vi "Write Table Predefined infos.vi"(0 "PDF Table Class.lvclass in":refnum<class "Pdfp Table Class.lvclass">, 5 "Predefined Borders":T19={"Borders"=0, "Header"={"Thickness"=1.0, "Line"=0, "Background "=16777226}, "Data"={"Thickness"=0.5, "Line"=0, "Background "=16777215}}, 7 "Borders IN":T21, 9 "Column Header format":T18, 11 "error in (no error)":errorcluster, 12 "Row Header format":T18, 13 "Datas format":T18) -> (4 "PDF Table Class.lvclass out":refnum<class "Pdfp Table Class.lvclass">, 8 "Row  [ ] OUT":T1, 15 "error out":errorcluster)   [LabVIEW 2019, in "Pdfp Table Class.lvclass"]
uses:
  <userlib>/Exaprom PDF/LV Class/Pdfp Table Class/Pdfp Table Class.lvclass
  <userlib>/Exaprom PDF/Controls/Table Controls/Simplified Table Row Borders [ ].ctl
  <userlib>/Exaprom PDF/Controls/Table Controls/Simplified Table Row Borders.ctl
  <userlib>/Exaprom PDF/Controls/Table Controls/Border and BG Color [ ].ctl
  <userlib>/Exaprom PDF/Controls/Table Controls/Border and BG Color.ctl
  <userlib>/Exaprom PDF/Controls/Table Controls/Cell Border 20 px.ctl
  <userlib>/Exaprom PDF/Controls/Table Controls/Row Predefined borders cluster.ctl
  <userlib>/Exaprom PDF/Controls/Table Controls/Row Predefined borders.ctl
  <userlib>/Exaprom PDF/Controls/Table Controls/Cell Font, type, Alignment and LS V2.ctl
  <userlib>/Exaprom PDF/Controls/Table Controls/Cell Type, Alignment and LS.ctl
  <userlib>/Exaprom PDF/Controls/Table Controls/Cell Alignment 20px.ctl
  <userlib>/Exaprom PDF/Controls/Table Controls/Text vertical arrangement.ctl
  <userlib>/Exaprom PDF/Controls/Text Controls/Line spacing.ctl
  <userlib>/Exaprom PDF/Controls/Font Controls/Font complete cluster.ctl
  <userlib>/Exaprom PDF/Controls/Font Controls/Font size.ctl
  <userlib>/Exaprom PDF/Controls/Font Controls/Font color.ctl
  <userlib>/Exaprom PDF/Controls/Font Controls/Type and encoding.ctl
  <userlib>/Exaprom PDF/Controls/Text Controls/Unicode/Type and run direction.ctl
  <userlib>/Exaprom PDF/Controls/Table Controls/Table Appearance and Font Row [ ].ctl
  <userlib>/Exaprom PDF/Controls/Table Controls/One Row Appearance.ctl
  <userlib>/Exaprom PDF/Controls/Table Controls/Row from to.ctl
  <userlib>/Exaprom PDF/Controls/Table Controls/Cell, Alignment, LS and Font - hide Vmerge.ctl
  <userlib>/Exaprom PDF/Controls/Table Controls/Cell Appearance.ctl
  <userlib>/Exaprom PDF/Controls/Table Controls/Merge Horizontal.ctl
  <userlib>/Exaprom PDF/Controls/Table Controls/Merge Vertical.ctl
  <userlib>/Exaprom PDF/LV Class/Pdfp Table Class/Pdfp Table Class.lvclass/Pdfp Table Class.ctl
  <userlib>/Exaprom PDF/Controls/Table Controls/Table Custom type Titles or Datas.ctl
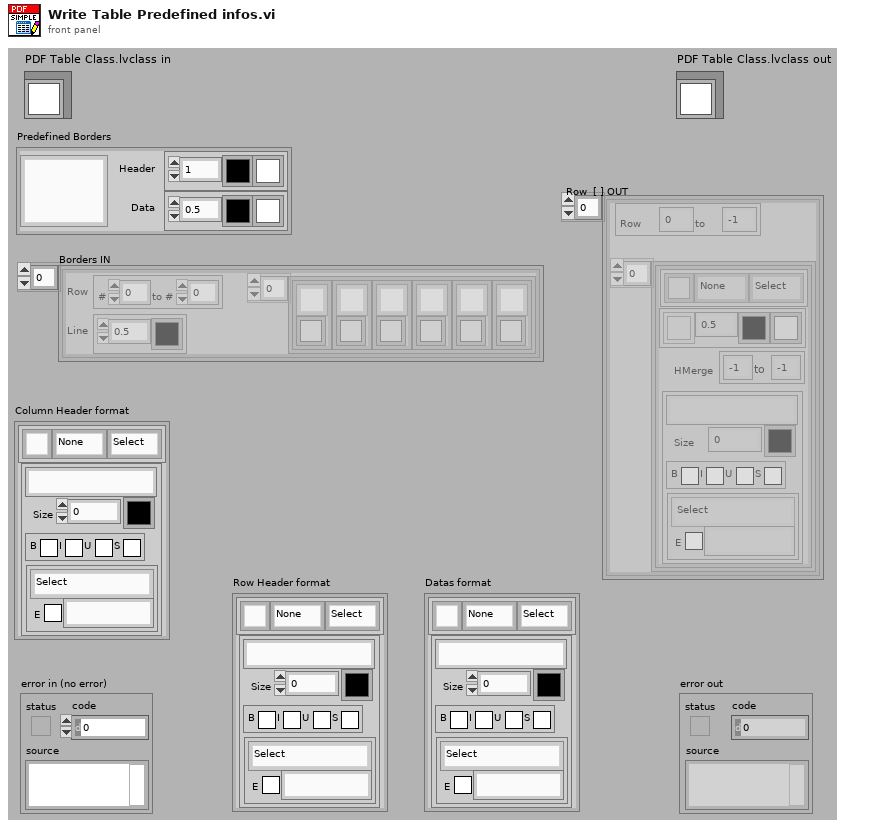
[diagram p1: front panel]
types:
  T1 = typedef "Table Appearance and Font Row [ ].ctl" = T2[]
  T2 = typedef "One Row Appearance.ctl" = cluster{"Row":T3, "Cell [ ]":T4[]}
  T3 = typedef "Row from to.ctl" = cluster{"From #":i16, "to #":i16}
  T4 = typedef "Cell, Alignment, LS and Font - hide Vmerge.ctl" = cluster{"Text":T5, "Cell Appearance":T9, "HMerge":T11, "VMerge":T12, "Font":T13}
  T5 = typedef "Cell Type, Alignment and LS.ctl" = cluster{"Cell Alignment":T6, "Text rotation":T7, "Line spacing":T8}
  T6 = typedef "Cell Alignment 20px.ctl" = u16
  T7 = typedef "Text vertical arrangement.ctl" = enum16{"None", "Clockwise", "Counterclockwise"}
  T8 = typedef "Line spacing.ctl" = enum16{"Select", "1.0", "1.5", "2.0"}
  T9 = typedef "Cell Appearance.ctl" = cluster{"Border":T10, "Thickness":sgl, "Color":u32, "BG":u32}
  T10 = typedef "Cell Border 20 px.ctl" = u16
  T11 = typedef "Merge Horizontal.ctl" = cluster{"From":i8, "to":i8}
  T12 = typedef "Merge Vertical.ctl" = cluster{"From":i8, "to":i8}
  T13 = typedef "Font complete cluster.ctl" = cluster{"Name":string, "Size":T14, "Color":T15, "Style":cluster{"Bold":bool, "Italic":bool, "Underline":bool, "Strikeout":bool}, "Type":T16}
  T14 = typedef "Font size.ctl" = sgl
  T15 = typedef "Font color.ctl" = u32
  T16 = typedef "Type and encoding.ctl" = cluster{"Type&direction":T17, "Embedded":bool, "Encoding":string}
  T17 = typedef "Type and run direction.ctl" = enum16{"Select", "ASCII", "UTF-16", "UTF-16 (default)", "UTF-16 (LTR)", "UTF-16 (RTL)"}
  T18 = typedef "Cell Font, type, Alignment and LS V2.ctl" = cluster{"Cell Type, Alignment and LS":T5, "Font":T13}
  T19 = typedef "Row Predefined borders cluster.ctl" = cluster{"Borders":T20, "Header":cluster{"Thickness":sgl, "Line":u32, "Background ":u32}, "Data":cluster{"Thickness":sgl, "Line":u32, "Background ":u32}}
  T20 = typedef "Row Predefined borders.ctl" = u16
  T21 = typedef "Simplified Table Row Borders [ ].ctl" = T22[]
  T22 = typedef "Simplified Table Row Borders.ctl" = cluster{"Row":cluster{"#":i16, "to #":i16}, "Line":cluster{"Thickness":sgl, "Color":u32}, "Column Borders [ ]":T23}
  T23 = typedef "Border and BG Color [ ].ctl" = T24[]
  T24 = typedef "Border and BG Color.ctl" = cluster{"Cell Border":T10, "BG":u32}
  T25 = typedef "Table Custom type Titles or Datas.ctl" = enum16{"Title", "Data"}
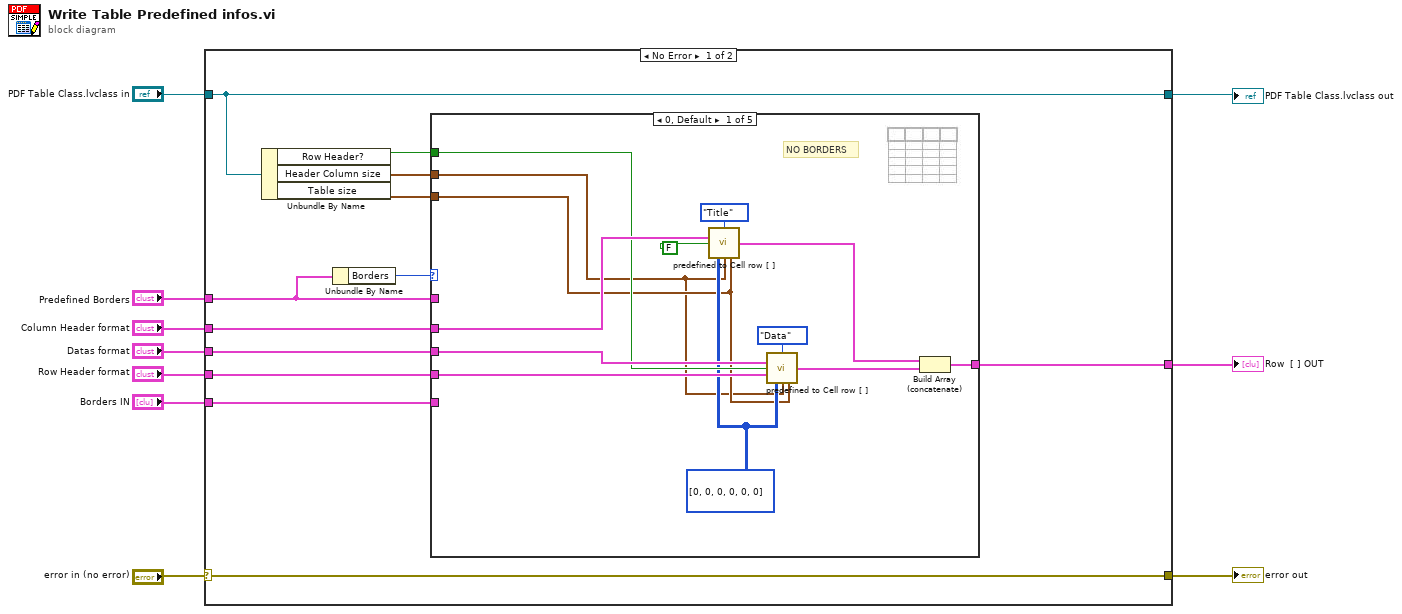
[diagram p0: block diagram]
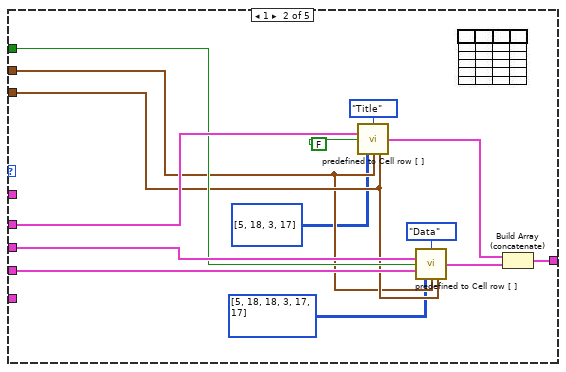
[diagram p2: hidden frame]
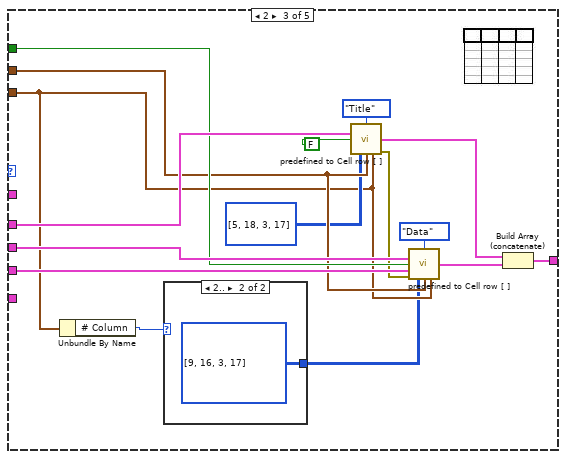
[diagram p3: hidden frame]
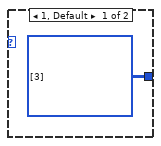
[diagram p4: hidden frame]
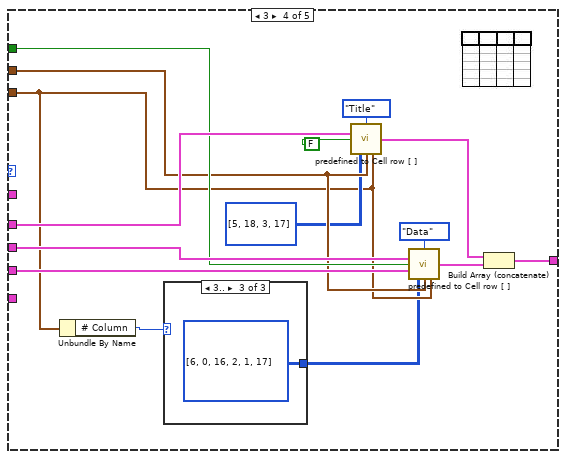
[diagram p5: hidden frame]
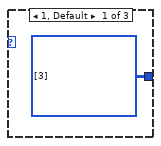
[diagram p6: hidden frame]
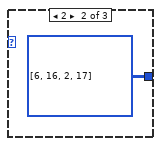
[diagram p7: hidden frame]
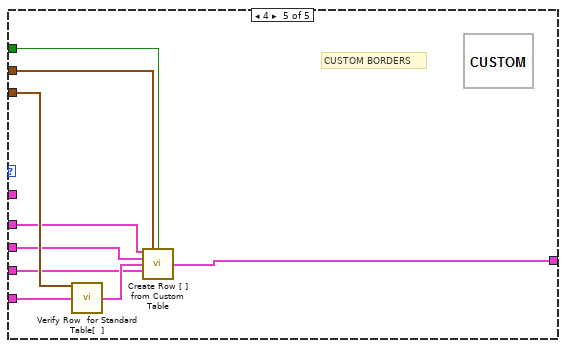
[diagram p8: hidden frame]
diagram:
  n1 = case shown="No Error" "error in (no error)" {
    selector: "error in (no error)" -> [w13 w96]
    tunnel: [w13 w96] -> w8
    tunnel: "Borders IN" -> [w22 _]
    tunnel: "Predefined Borders" -> [w21 _]
    tunnel: "PDF Table Class.lvclass in" -> [w12 w95]
    tunnel: [w12 w95] -> w5
    tunnel: "Column Header format" -> [w19 _]
    tunnel: "Row Header format" -> [w18 _]
    tunnel: "Datas format" -> [w17 _]
    tunnel: [w11 _] -> w1
    frame No Error {
      n2 = Unbundle By Name(w12) -> ("Row Header?"=w16:bool, "Header Column size"=w15:cluster{"# Column":u16, "# Row":u16}, "Table size"=w14:cluster{"# Column":u16, "# Row":u16})
      n3 = Unbundle By Name(w21) -> ("Borders"=w20:T20)
      n4 = case shown="0, Default" w20 {
        tunnel: w22 -> [_ _ _ _ w94]
        tunnel: w21 -> [_ _ _ _ _]
        tunnel: [w35 w49 w65 w82 w86] -> w11
        tunnel: w19 -> [w32 w46 w62 w79 w90]
        tunnel: w18 -> [w30 w44 w60 w77 w87]
        tunnel: w17 -> [w29 w43 w59 w76 w89]
        tunnel: w16 -> [w28 w42 w58 w75 w92]
        tunnel: w15 -> [w23 w38 w55 w72 w91]
        tunnel: w14 -> [w24 w39 w53 w70 w93]
        frame 0, Default {
          w27 = T10[][] [[0, 0, 0], [0, 0, 0]] ("Title tous 2")
          # "NO BORDERS"
          n5 = call <userlib>:"predefined to Cell row [ ].vi"("Titles or datas"=Table_Custom_type_Titles_or_Datas."Title", "Format Column Header or Data"=w32, "Row Header?"=FALSE, "Title tous"=w27, "Header Column size"=w23, "Table size"=w24) -> ("Row  [ ]"=w25:T1)  [unwired: 4 in, 5 out]
          n6 = call <userlib>:"predefined to Cell row [ ].vi"("Titles or datas"=Table_Custom_type_Titles_or_Datas."Data", "Format Column Header or Data"=w29, "Row Header?"=w28, "Format Row Header"=w30, "Title tous"=w27, "Header Column size"=w23, "Table size"=w24) -> ("Row  [ ]"=w26:T1)  [unwired: 3 in, 5 out]
          n7 = Build Array (concatenate)(w25, w26) -> (w35:T1)
        }
        frame 1 {
          n8 = call <userlib>:"predefined to Cell row [ ].vi"("Titles or datas"=Table_Custom_type_Titles_or_Datas."Title", "Format Column Header or Data"=w46, "Row Header?"=FALSE, "Title tous"=T10[][] [[5, 18], [3, 17]], "Header Column size"=w38, "Table size"=w39) -> ("Row  [ ]"=w40:T1)  [unwired: 4 in, 5 out]
          n9 = call <userlib>:"predefined to Cell row [ ].vi"("Titles or datas"=Table_Custom_type_Titles_or_Datas."Data", "Format Column Header or Data"=w43, "Row Header?"=w42, "Format Row Header"=w44, "Title tous"=T10[][] [[5, 18, 18], [3, 17, 17]] ("Array 7"), "Header Column size"=w38, "Table size"=w39) -> ("Row  [ ]"=w41:T1)  [unwired: 3 in, 5 out]
          n10 = Build Array (concatenate)(w40, w41) -> (w49:T1)
        }
        frame 2 {
          n11 = Unbundle By Name(w53) -> ("# Column"=w52:u16)
          n12 = case shown="2.." w52 {
            tunnel: [T10[][] [[3]] ("Data 1 x1") T10[][] [[9, 16], [3, 17]] ("Array 9")] -> w51
            frame 1, Default {
            }
            frame 2.. {
            }
          }
          n13 = call <userlib>:"predefined to Cell row [ ].vi"("Titles or datas"=Table_Custom_type_Titles_or_Datas."Title", "Format Column Header or Data"=w62, "Row Header?"=FALSE, "Title tous"=T10[][] [[5, 18], [3, 17]], "Header Column size"=w55, "Table size"=w53) -> ("Row  [ ]"=w56:T1, "error duplicate"=w50:errorcluster)  [unwired: 4 in, 4 out]
          n14 = call <userlib>:"predefined to Cell row [ ].vi"("Titles or datas"=Table_Custom_type_Titles_or_Datas."Data", "Format Column Header or Data"=w59, "Row Header?"=w58, "Format Row Header"=w60, "error in (no error)"=w50, "Title tous"=w51, "Header Column size"=w55, "Table size"=w53) -> ("Row  [ ]"=w57:T1)  [unwired: 2 in, 5 out]
          n15 = Build Array (concatenate)(w56, w57) -> (w65:T1)
        }
        frame 3 {
          n16 = Unbundle By Name(w70) -> ("# Column"=w69:u16)
          n17 = case shown="3.." w69 {
            tunnel: [T10[][] [[3]] ("Data 1 x1") T10[][] [[6, 16], [2, 17]] ("Array 13") T10[][] [[6, 0, 16], [2, 1, 17]] ("Array 14")] -> w68
            frame 1, Default {
            }
            frame 2 {
            }
            frame 3.. {
            }
          }
          n18 = call <userlib>:"predefined to Cell row [ ].vi"("Titles or datas"=Table_Custom_type_Titles_or_Datas."Title", "Format Column Header or Data"=w79, "Row Header?"=FALSE, "Title tous"=T10[][] [[5, 18], [3, 17]], "Header Column size"=w72, "Table size"=w70) -> ("Row  [ ]"=w73:T1)  [unwired: 4 in, 5 out]
          n19 = call <userlib>:"predefined to Cell row [ ].vi"("Titles or datas"=Table_Custom_type_Titles_or_Datas."Data", "Format Column Header or Data"=w76, "Row Header?"=w75, "Format Row Header"=w77, "Title tous"=w68, "Header Column size"=w72, "Table size"=w70) -> ("Row  [ ]"=w74:T1)  [unwired: 3 in, 5 out]
          n20 = Build Array (concatenate)(w73, w74) -> (w82:T1)
        }
        frame 4 {
          # "CUSTOM BORDERS"
          n21 = call <userlib>:"Verify Row  for Standard Table[  ].vi"("Table size"=w93, "Borders IN"=w94) -> ("Borders OUT"=w88:T21)  [unwired: 13 in]
          n22 = call <userlib>:"Create Row [ ] from Custom Table.vi"("Column Header format"=w90, "Header Column size"=w91, "Row Header?"=w92, "Datas format"=w89, "Borders IN"=w88, "Row Header format"=w87) -> ("Row  [ ] OUT"=w86:T1)  [unwired: 9 in]
        }
      }
    }
    frame Error {
    }
  }
  "error out" <- w8
  "PDF Table Class.lvclass out" <- w5
  "Row  [ ] OUT" <- w1
